vi "FilterLittle.vi"(9 "timeout in ms":i32=50, 10 "Little Boat Queues":T2, 11 "NotifierReff":T1) -> ()   [LabVIEW 2013]
doc: "This code takes values that were written to HB queues and sends those to the notifiers for the MB and FB. Basic filtering can be done here. For example, the GPS and compass data does not get written to the notifiers if it is invalid.\n\nEric Schneider, April 2014"
uses:
  Data/TypeDefs/UTM Location.ctl
  Data/TypeDefs/Notifiers.ctl
  Data/TypeDefs/Sail Set Suggestions.ctl
  Data/TypeDefs/Rudder Set Suggestions.ctl
  Data/TypeDefs/OverrideInformation.ctl
  Data/TypeDefs/OverrideMode.ctl
  Data/TypeDefs/MotorSetup.ctl
  Data/TypeDefs/DynamixelSetupInfo.ctl
  Data/TypeDefs/AirmarStatus.ctl
  Data/TypeDefs/HardwareOnline.ctl
  Data/TypeDefs/DynamixelCycleTracker.ctl
  Data/TypeDefs/RC Input Values.ctl
  Classes/Missions/GenericMission/GenericMission.lvclass
  Classes/Waypoint/Waypoint.lvclass
  Utilities/Math/Angles/Angle/Angle.lvclass
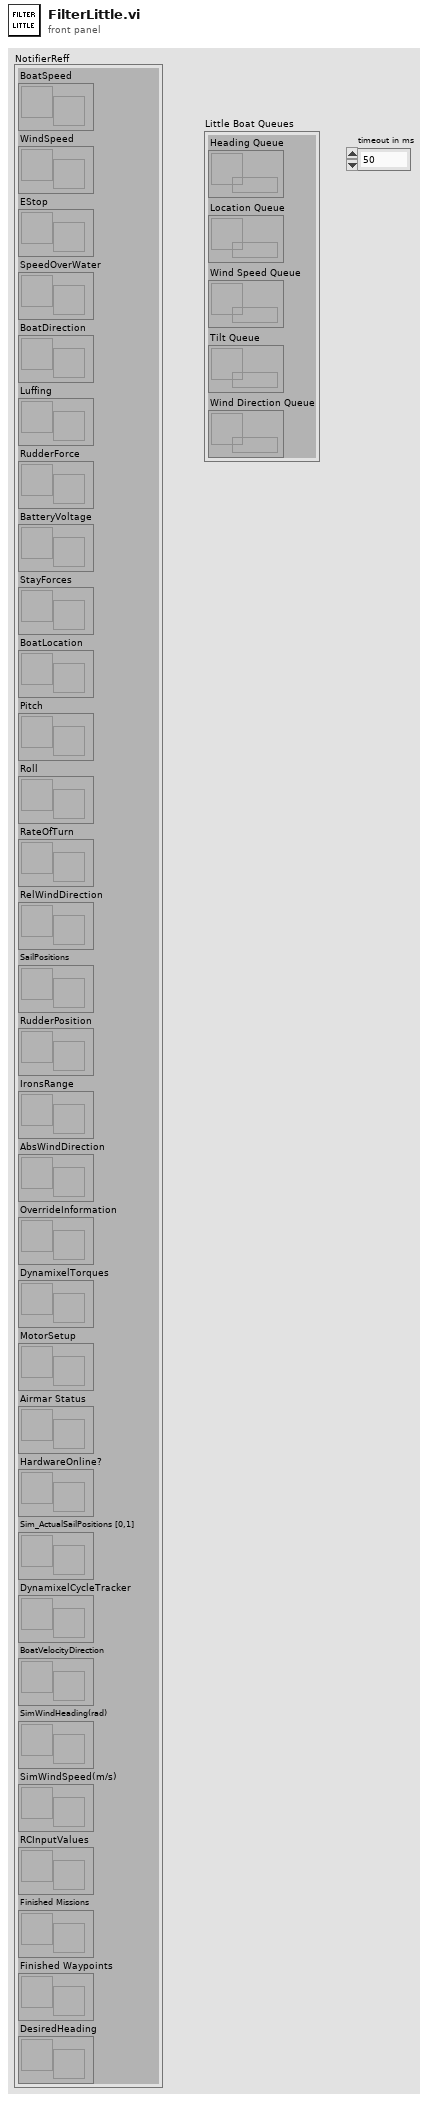
[diagram p1: front panel]
types:
  T1 = typedef "Notifiers.ctl" = cluster{"BoatSpeed":refnum<notifier>, "WindSpeed":refnum<notifier>, "EStop":refnum<notifier>, "SpeedOverWater":refnum<notifier>, "BoatDirection":refnum<notifier>, "Luffing":refnum<notifier>, "RudderForce":refnum<notifier>, "BatteryVoltage":refnum<notifier>, "StayForces":refnum<notifier>, "BoatLocation":refnum<notifier>, "Pitch":refnum<notifier>, "Roll":refnum<notifier>, "RateOfTurn":refnum<notifier>, "RelWindDirection":refnum<notifier>, "SailPositions":refnum<notifier>, "RudderPosition":refnum<notifier>, "IronsRange":refnum<notifier>, "AbsWindDirection":refnum<notifier>, "OverrideInformation":refnum<notifier>, "DynamixelTorques":refnum<notifier>, "MotorSetup":refnum<notifier>, "Airmar Status":refnum<notifier>, "HardwareOnline?":refnum<notifier>, "Sim_ActualSailPositions [0,1]":refnum<notifier>, "DynamixelCycleTracker":refnum<notifier>, "BoatVelocityDirection":refnum<notifier>, "SimWindHeading(rad)":refnum<notifier>, "SimWindSpeed(m/s)":refnum<notifier>, "RCInputValues":refnum<notifier>, "Finished Missions":refnum<notifier>, "Finished Waypoints":refnum<notifier>, "DesiredHeading":refnum<notifier>}
  T2 = cluster{"Heading Queue":refnum<queue>, "Location Queue":refnum<queue>, "Wind Speed Queue":refnum<queue>, "Tilt Queue":refnum<queue>, "Wind Direction Queue":refnum<queue>}
  T3 = typedef "UTM Location.ctl" = cluster{"UTM Zone":dbl, "Hemisphere":enum16{"North", "South"}, "East":dbl, "North":dbl}
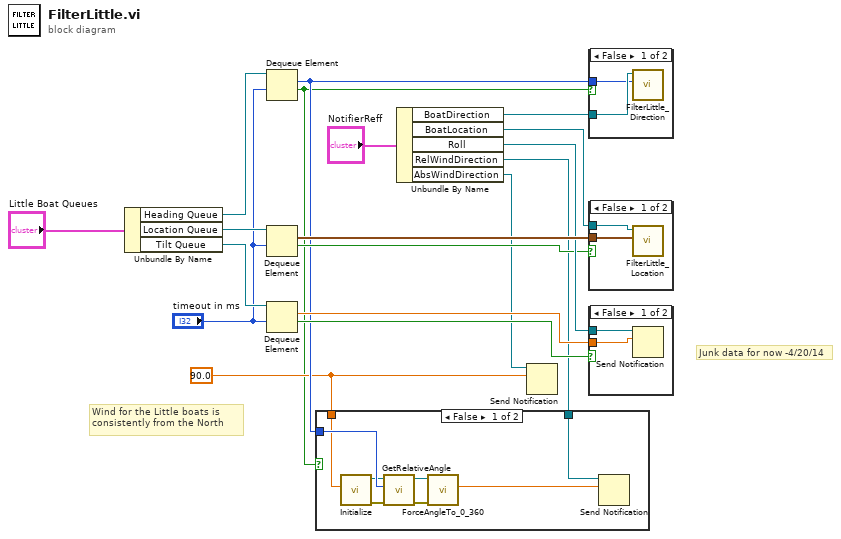
[diagram p0: block diagram]
diagram:
  w2 = 90.0 ("notification")
  # "Junk data for now -4/20/14"
  # "Wind for the Little boats is consistently from the North"
  n1 = Unbundle By Name("Little Boat Queues") -> ("Heading Queue"=w15:refnum<queue>, "Location Queue"=w13:refnum<queue>, "Tilt Queue"=w12:refnum<queue>)
  n2 = Dequeue Element(queue=w15, timeout in ms (-1)="timeout in ms") -> (element=w3:i32, timed out?=w1:bool)  [unwired: 1 in, 2 out]
  n3 = Dequeue Element(queue=w13, timeout in ms (-1)="timeout in ms") -> (element=w14:T3, timed out?=w7:bool)  [unwired: 1 in, 2 out]
  n4 = Dequeue Element(queue=w12, timeout in ms (-1)="timeout in ms") -> (element=w11:dbl, timed out?=w8:bool)  [unwired: 1 in, 2 out]
  n5 = Unbundle By Name("NotifierReff") -> ("BoatDirection"=w16:refnum<notifier>, "BoatLocation"=w6:refnum<notifier>, "Roll"=w10:refnum<notifier>, "RelWindDirection"=w4:refnum<notifier>, "AbsWindDirection"=w5:refnum<notifier>)
  n6 = case shown="False" w1 {
    tunnel: w4 -> [w24 _]
    tunnel: w3 -> [w23 _]
    tunnel: w2 -> [w21 _]
    frame False {
      n7 = call "Initialize.vi"("Input Angle (Deg.)"=w21) -> ("error out"=w25:errorcluster, "Angle out"=w22:refnum<class "Angle.lvclass">)  [unwired: 9 in]
      n8 = call "GetRelativeAngle.vi"("error in (no error)"=w25, "Boat Heading (Deg.)"=w23, "Angle in"=w22) -> ("error out"=w19:errorcluster, "Relative Angle"=w20:refnum<class "Angle.lvclass">)  [unwired: 6 in, 1 out]
      n9 = call "ForceAngleTo_0_360.vi"("error in (no error)"=w19, "Angle in"=w20) -> ("Relative Angle"=w26:dbl)  [unwired: 8 in, 1 out]
      n10 = Send Notification(notification=w26, notifier=w24) -> ()  [unwired: 1 in, 2 out]
    }
    frame True {
    }
  }
  n11 = Send Notification(notification=w2, notifier=w5) -> ()  [unwired: 1 in, 2 out]
  n12 = case shown="False" w1 {
    tunnel: w16 -> [w28 _]
    tunnel: w3 -> [w27 _]
    frame False {
      n13 = call "FilterLittle_Direction.vi"("Numeric"=w27, "Notifier in"=w28) -> ()  [unwired: 10 in]
    }
    frame True {
    }
  }
  n14 = case shown="False" w7 {
    tunnel: w14 -> [w30 _]
    tunnel: w6 -> [w29 _]
    frame False {
      n15 = call "FilterLittle_Location.vi"("UTM Location"=w30, "Notifier in"=w29) -> ()  [unwired: 10 in]
    }
    frame True {
    }
  }
  n16 = case shown="False" w8 {
    tunnel: w11 -> [w32 _]
    tunnel: w10 -> [w31 _]
    frame False {
      n17 = Send Notification(notification=w32, notifier=w31) -> ()  [unwired: 1 in, 2 out]
    }
    frame True {
    }
  }
